vi "pace pluse measurement_mso7014b.vi"(8 "error in (no error)":errorcluster, 11 "VISA resource name":refnum<visa-resource-name>) -> (0 "CH3 Waveform":waveform(dbl)(graph), 1 "CH1 Waveform":waveform(dbl)(graph), 2 "添加的数组":waveform(dbl)[](array[waveform]), 3 "Pluse Frequency":dbl, 5 "Pluse Interval":dbl)   [LabVIEW 2016]
uses:
  <instrlib>/Agilent 6000 Series/Agilent 6000 Series.lvlib
panel:
  out "VISA resource name out":refnum<visa-resource-name>
  out "error out":errorcluster
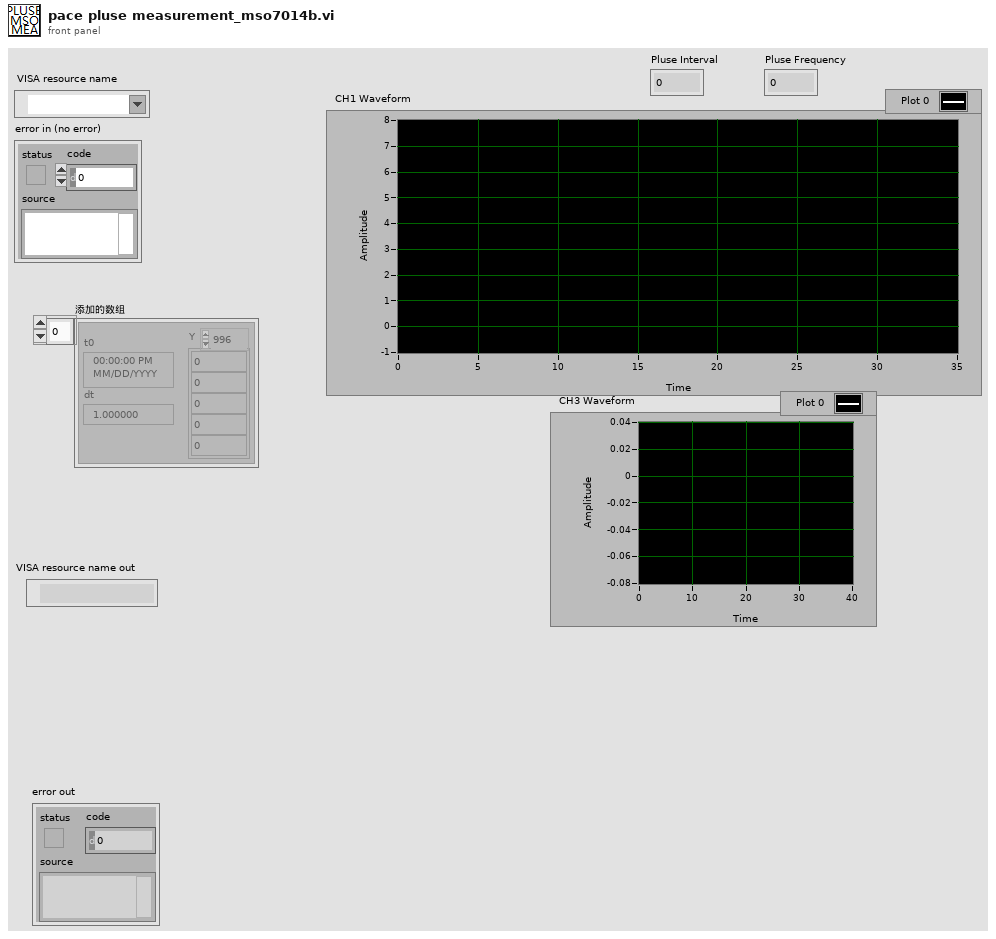
[diagram p1: front panel]
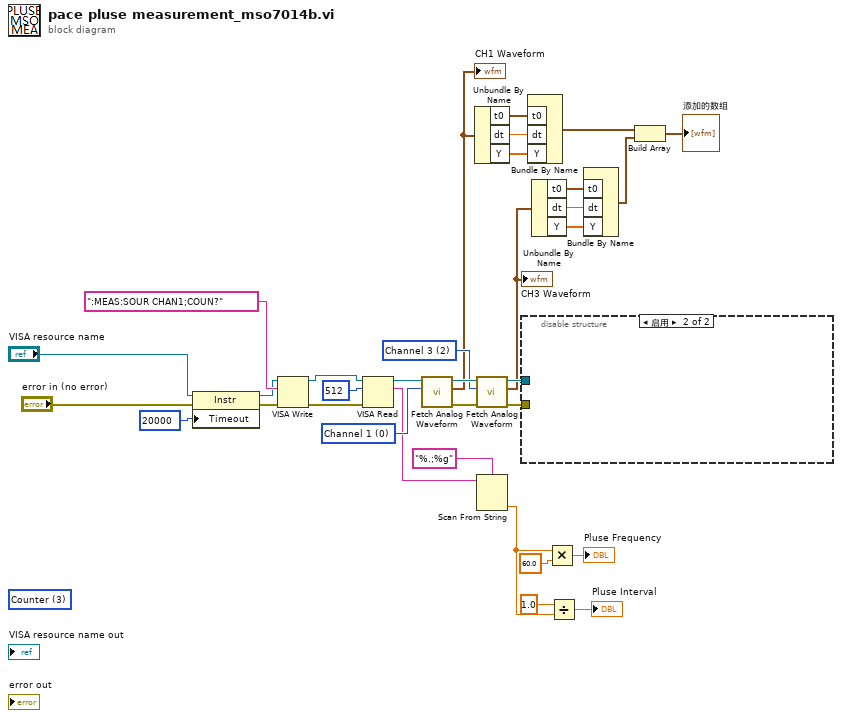
[diagram p0: block diagram]
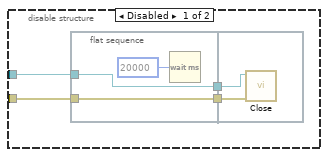
[diagram p2: hidden frame]
diagram:
  (unwired) u16 3 items=["Amplitude", "Voltage Average", "Base", "Counter", "Delay", "Duty Cycle", "Fall Time", "Frequency", "Voltage Max", "Voltage Min", "Overshoot", "Voltage Vpp", "Period", "Phase", "Preshoot", "Rise Time", "Voltage RMS", "Top", "Width Positive", "X at Max Y", "X at Min Y"] ("Measurement Function (7: Frequency)")
  w32 = u16 2 items=["Channel 1", "Channel 2", "Channel 3", "Channel 4", "Math"] ("Source (0: Channel 1)")
  w34 = u16 0 items=["Channel 1", "Channel 2", "Channel 3", "Channel 4", "Math"] ("Source (0: Channel 1)")
  n1 = property class="Instr"(reference="VISA resource name", error in="error in (no error)", "Timeout"=u32 20000 ("General Settings:Timeout Value")) -> (reference out=w6:refnum<visa-resource-name>, error out=w4:errorcluster)
  n2 = VISA Write(VISA resource name=w6, write buffer=":MEAS:SOUR CHAN1;COUN?" ("写入缓冲区"), error in (no error)=w4) -> (VISA resource name out=w14:refnum<visa-resource-name>, error out=w15:errorcluster)  [unwired: 1 out]
  n3 = VISA Read(VISA resource name=w14, byte count=u32 512, error in (no error)=w15) -> (VISA resource name out=w10:refnum<visa-resource-name>, read buffer=w11:string)  [unwired: 2 out]
  n4 = call <instrlib>:"Fetch Analog Waveform.vi"("Source (0: Channel 1)"=w34, "VISA resource name"=w10) -> ("error out"=w29:errorcluster, "Waveform Data"=w28:waveform(dbl), "VISA resource name out"=w33:refnum<visa-resource-name>)  [unwired: 7 in]
  "CH1 Waveform" <- w28
  n5 = Unbundle By Name(w28) -> ("t0"=w27:timestamp, "dt"=w26:dbl, "Y"=w25:dbl[])
  n6 = call <instrlib>:"Fetch Analog Waveform.vi"("error in (no error)"=w29, "Source (0: Channel 1)"=w32, "VISA resource name"=w33) -> ("error out"=w30:errorcluster, "Waveform Data"=w21:waveform(dbl), "VISA resource name out"=w31:refnum<visa-resource-name>)  [unwired: 6 in]
  "CH3 Waveform" <- w21
  n7 = Scan From String(format string="%.;%g", input string=w11) -> (output 1=w3:dbl)  [unwired: 3 in, 3 out]
  n8 = disable-structure shown="启用" {
    disable-tunnel: w31 -> [w36 _]
    disable-tunnel: w30 -> [w35 _]
    frame Disabled {
      n9 = flat-sequence {
        tunnel: w35 -> [w40]
        tunnel: w36 -> [w41]
        tunnel: [w41] -> w38
        tunnel: [w40] -> w37
        tunnel: w38 -> [w43]
        tunnel: w37 -> [w42]
        frame #0 {
          n10 = Wait (ms)(milliseconds to wait=u32 20000 ("等待时间（毫秒）")) -> ()  [unwired: 1 out]
        }
        frame #1 {
          n11 = call <instrlib>:"Close.vi"("error in (no error)"=w42, "VISA resource name"=w43) -> ()  [unwired: 9 in, 1 out]
        }
      }
    }
    frame Enabled {
    }
  }
  n12 = Bundle By Name("t0"=w27, "dt"=w26, "Y"=w25) -> (w20:waveform(dbl))  [unwired: 1 in]
  n13 = Unbundle By Name(w21) -> ("t0"=w22:timestamp, "dt"=w23:dbl, "Y"=w24:dbl[])
  n14 = Multiply(x=w3, y=60.0) -> (x*y=→"Pluse Frequency":dbl)
  n15 = Divide(x=1.0, y=w3) -> (x/y=→"Pluse Interval":dbl)
  n16 = Bundle By Name("t0"=w22, "dt"=w23, "Y"=w24) -> (w19:waveform(dbl))  [unwired: 1 in]
  n17 = Build Array(w20, w19) -> (→"添加的数组":waveform(dbl)[])
